vi "test2.vi"   [LabVIEW 2021]
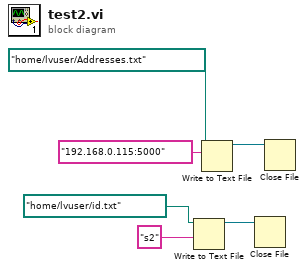
[diagram p0: block diagram]
diagram:
  n1 = Write to Text File(file (use dialog)=path "/home/lvuser/id.txt" ("file path (use dialog)"), text="s2") -> (refnum out=w3:refnum<file>)  [unwired: 2 in, 2 out]
  n2 = Write to Text File(file (use dialog)=path "/home/lvuser/Addresses.txt" ("file path (use dialog)"), text="192.168.0.115:5000") -> (refnum out=w4:refnum<file>)  [unwired: 2 in, 2 out]
  n3 = Close File(refnum=w3) -> ()  [unwired: 1 in, 2 out]
  n4 = Close File(refnum=w4) -> ()  [unwired: 1 in, 2 out]
